vi "addNode.vi"(0 "reference":refnum<class "SystemNode.lvclass">, 1 "node":refnum<class "AbstractNode.lvclass">, 2 "point2D":T1 {"y" format="%.2f"; "x" format="%.2f"}, 5 "error in (no error)":errorcluster) -> (14 "reference out":refnum<class "SystemNode.lvclass">, 15 "added":bool, 19 "error out":errorcluster)   [LabVIEW 2020, in "SystemNode.lvclass"]
doc: "public boolean addNode(Node n, Point2D p)"
uses:
  <resource>/Framework/Providers/Open_GDS/UML/SystemNode_class/SystemNode.lvclass
  <resource>/Framework/Providers/Open_GDS/UML/AbstractNode_class/AbstractNode.lvclass
  <resource>/Framework/Providers/Open_GDS/UML/General/Point/Point Point2D.ctl
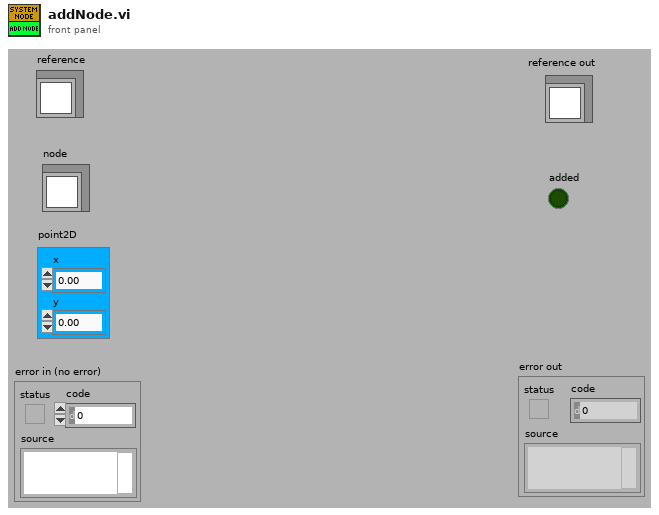
[diagram p1: front panel]
types:
  T1 = typedef "Point Point2D.ctl" = cluster{"x":dbl, "y":dbl}
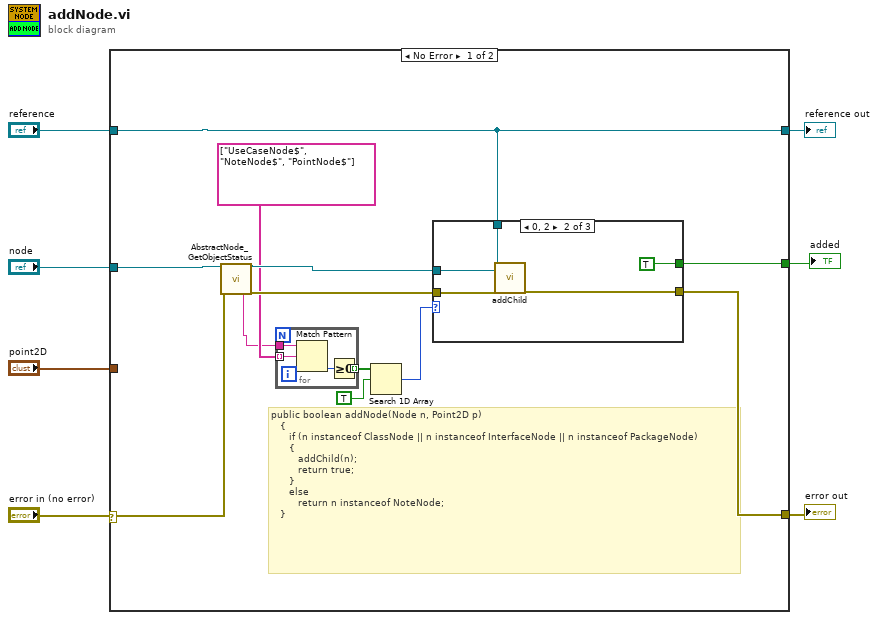
[diagram p0: block diagram]
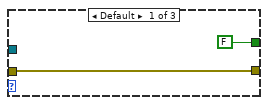
[diagram p2: hidden frame]
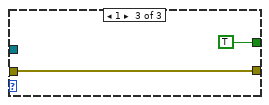
[diagram p3: hidden frame]
diagram:
  n1 = case shown="No Error" "error in (no error)" {
    selector: "error in (no error)" -> [w9 w33]
    tunnel: "reference" -> [w18 w34]
    tunnel: [w16 w33] -> w6
    tunnel: [w18 w34] -> w5
    tunnel: "node" -> [w19 _]
    tunnel: "point2D" -> [_ _]
    tunnel: [w17 _] -> w1
    frame No Error {
      # "public boolean addNode(Node n, Point2D p)\n   {\n      if (n instanceof ClassNode || n instanceof InterfaceNode || n instanceof PackageNode)\n      {\n         addChild(n);\n         return true;\n      }\n      else\n         return n instanceof NoteNode;\n   }"
      n2 = call <resource>:"AbstractNode_GetObjectStatus.vi"("reference in"=w19, "error in (no error)"=w9) -> ("Class name"=w8:string, "reference out"=w14:refnum<class "AbstractNode.lvclass">, "error out"=w15:errorcluster)  [unwired: 15 out]
      n3 = for {
        tunnel: w8 -> [w23]
        tunnel: string[] ["UseCaseNode$", "NoteNode$", "PointNode$"] -> [w22] mode=indexing
        tunnel: [w20] -> w12 mode=indexing
        n4 = Match Pattern(string=w23, regular expression=w22) -> (offset past match=w21:i32)  [unwired: 4 out]
        n5 = Greater Or Equal To 0?(x=w21) -> (x >= 0?=w20:bool)
      }
      n6 = Search 1D Array(1D array=w12, element=TRUE) -> (index of element=w10:i32)  [unwired: 1 out]
      n7 = case shown="0, 2" w10 {
        tunnel: [FALSE TRUE TRUE] -> w17
        tunnel: w15 -> [w24 w29 w32]
        tunnel: [w24 w26 w32] -> w16
        tunnel: w18 -> [_ w28 _]
        tunnel: w14 -> [_ w27 _]
        frame Default {
        }
        frame 0, 2 {
          n8 = call-dynamic "addChild.vi"("reference"=w28, "node"=w27, "error in (no error)"=w29) -> ("error out"=w26:errorcluster)  [unwired: 15 in, 1 out]
        }
        frame 1 {
        }
      }
    }
    frame Error {
    }
  }
  "reference out" <- w5
  "error out" <- w6
  "added" <- w1
